vi "Cmd.ReadRegisteredString.Vi"(6 "Timeout [ms] (1000)":i32=1000, 8 "error in":errorcluster, 9 "LineNo":u8=1 min=1 max=16, 10 "ToolNo":u16=100 min=100 max=499, 11 "cID in":refnum<k5>) -> (0 "error out":errorcluster, 2 "RegisteredString":string, 3 "cID out":refnum<k5>)   [LabVIEW 2016]
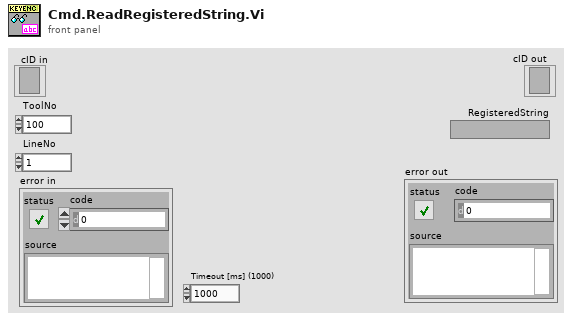
[diagram p1: front panel]
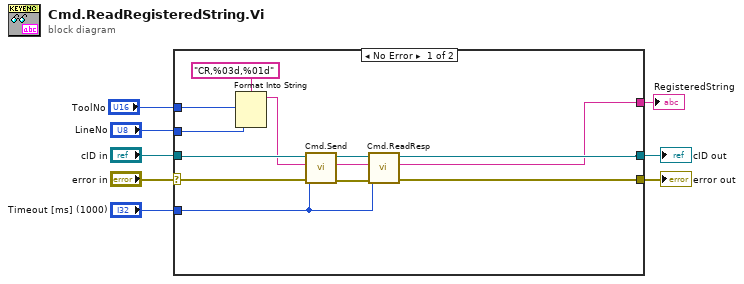
[diagram p0: block diagram]
diagram:
  n1 = case shown="No Error" "error in" {
    selector: "error in" -> [w19 w21]
    tunnel: "Timeout [ms] (1000)" -> [w14 _]
    tunnel: "cID in" -> [w20 w22]
    tunnel: [w13 w22] -> w5
    tunnel: [w12 w21] -> w4
    tunnel: "LineNo" -> [w11 _]
    tunnel: "ToolNo" -> [w10 _]
    tunnel: [w9 _] -> w1
    frame No Error {
      n2 = Format Into String(format string="CR,%03d,%01d", w10, w11) -> (resulting string=w16:string)  [unwired: 2 in, 1 out]
      n3 = call "Cmd.Send.vi"("error in (no error)"=w19, "Timeout [ms] (1000)"=w14, "Command"=w16, "connection ID"=w20) -> ("error out"=w15:errorcluster, "connection ID out"=w17:refnum<k5>)  [unwired: 6 in]
      n4 = call "Cmd.ReadResp.vi"("error in (no error)"=w15, "Timeout [ms] (1000)"=w14, "Request"=w16, "connection ID"=w17) -> ("error out"=w12:errorcluster, "ResponseParameters"=w9:string, "connection ID out"=w13:refnum<k5>)  [unwired: 5 in]
    }
    frame Error {
    }
  }
  "cID out" <- w5
  "error out" <- w4
  "RegisteredString" <- w1
